vi "Teleop.vi"(10 "Match Info":T1={"Autonomous Elapsed Seconds"=0.0, "TeleOp Elapsed Seconds"=0.0, "Disabled Elapsed Seconds"=0.0, "Visited Autonomous"=FALSE, "Visited TeleOp"=FALSE, "Visited Disabled"=FALSE, "Autonomous Settings"={"Autonomous Style"=enum."Independent", "VI Refnum"=refnum}}, 11 "Call Context":T2) -> ()   [LabVIEW 2020]
doc: "This VI is called for each enabled TeleOp packet received from the DS. It is typically used to read from joysticks and other inputs and update I/O or setpoints for timed control loops. It should complete and return within 20 milliseconds or risk missing DS packets."
uses:
  <vilib>/Rock Robotics/WPI/DriverStation/WPI_DriverStationDerivedRobotMode.ctl
  <vilib>/Rock Robotics/WPI/DriverStation/WPI_DriverStationMatch Info.ctl
  Framework/Robot Global Data.vi
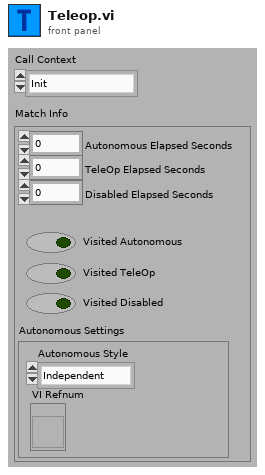
[diagram p1: front panel]
types:
  T1 = typedef "WPI_DriverStationMatch Info.ctl" = cluster{"Autonomous Elapsed Seconds":dbl, "TeleOp Elapsed Seconds":dbl, "Disabled Elapsed Seconds":dbl, "Visited Autonomous":bool, "Visited TeleOp":bool, "Visited Disabled":bool, "Autonomous Settings":cluster{"Autonomous Style":enum16{"Iterative", "Independent"}, "VI Refnum":refnum<vi>}}
  T2 = typedef "WPI_DriverStationDerivedRobotMode.ctl" = enum16{"Init", "Execute", "Stop"}
  T3 = typedef "Command Status Info.ctl" = cluster{"Name":string, "Status":T4, "notifier out":T5}
  T4 = typedef "Completion Status.ctl" = enum16{"Successful", "Aborted", "Incomplete"}
  T5 = typedef "Completion Notifier.ctl" = refnum<notifier>
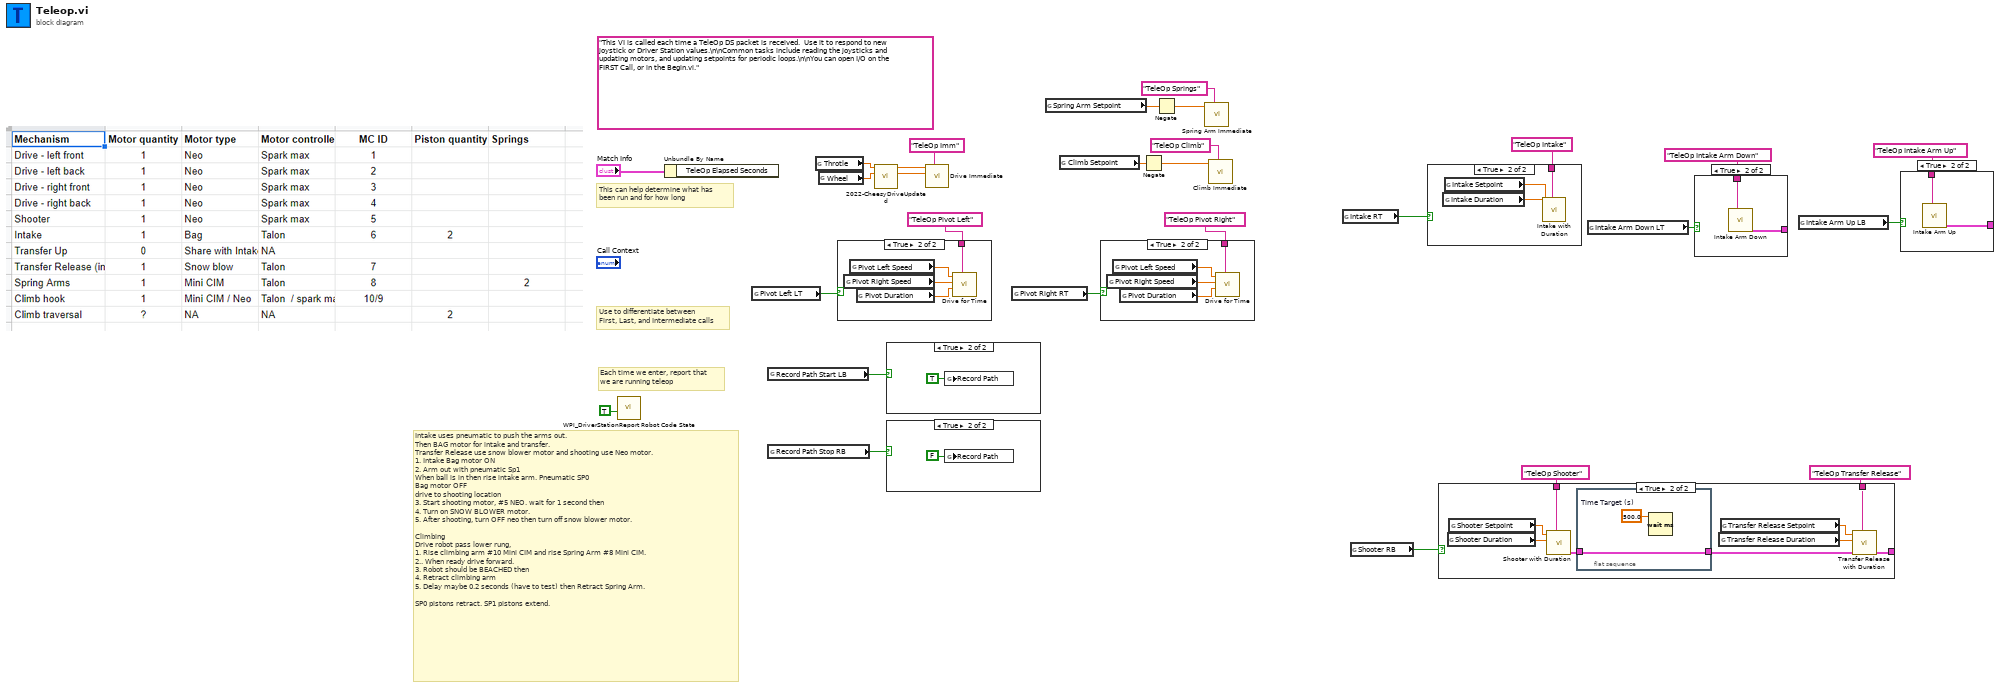
[diagram p0: block diagram]
diagram:
  (unwired) "This VI is called each time a TeleOp DS packet is received.  Use it to respond to new joystick or Driver Station values.\n\nCommon tasks include reading the joysticks and updating motors, and updating setpoints for periodic loops.\n\nYou can open I/O on the FIRST Call, or in the Begin.vi."
  # "Intake uses pneumatic to push the arms out. \nThen BAG motor for intake and transfer. \nTransfer Release use snow blower motor and shooting use Neo motor.\n1. Intake Bag motor ON\n2. Arm out with pneumatic Sp1\nWhen ball is in then rise intake arm. Pneumatic SP0\nBag motor OFF\ndrive to shooting location \n3. Start shooting motor, #5 NEO. wait for 1 second then\n4. Turn on SNOW BLOWER motor. \n5. After shooting, turn OFF neo then turn off snow blower motor.\n\nClimbing \nDrive robot pass lower rung, \n1. Rise climbing arm #10 Mini CIM and rise Spring Arm #8 Mini CIM. \n2.. When ready drive forward. \n3. Robot should be BEACHED then\n4. Retract climbing arm\n5. Delay maybe 0.2 seconds (have to test) then Retract Spring Arm.\n\nSP0 pistons retract. SP1 pistons extend."
  # "Each time we enter, report that\nwe are running teleop"
  # "Use to differentiate between\nFirst, Last, and Intermediate calls"
  # "This can help determine what has\nbeen run and for how long"
  n1 = call <vilib>:"WPI_DriverStationReport Robot Code State.vi"("TeleOp"=TRUE ("Autonomous")) -> ()  [unwired: 10 in, 1 out]
  n2 = Unbundle By Name("Match Info") -> ()  [unwired: 1 out]
  n3 = global read "Robot Global Data.vi" "Pivot Left LT"() -> (w5:bool)
  n4 = global read "Robot Global Data.vi" "Record Path Start LB"() -> (w2:bool)
  n5 = global read "Robot Global Data.vi" "Record Path Stop RB"() -> (w1:bool)
  n6 = global read "Robot Global Data.vi" "Throtle"() -> (w23:dbl)
  n7 = global read "Robot Global Data.vi" "Wheel"() -> (w22:dbl)
  n8 = case shown="True" w5 {
    tunnel: "TeleOp Pivot Left" ("Description") -> [_ w32]
    frame False {
    }
    frame True {
      n9 = global read "Robot Global Data.vi" "Pivot Right Speed"() -> (w30:dbl)
      n10 = global read "Robot Global Data.vi" "Pivot Left Speed"() -> (w31:dbl)
      n11 = global read "Robot Global Data.vi" "Pivot Duration"() -> (w29:dbl)
      n12 = call "Drive for Time.vi"("Description"=w32, "Seconds"=w29, "Right Speed"=w30, "Left Speed"=w31) -> ()  [unwired: 7 in, 1 out]
    }
  }
  n13 = call "2022-CheesyDriveUpdated.vi"("Throttle"=w23, "Wheel"=w22) -> ("Left PWM"=w25:dbl, "Right PWM"=w24:dbl)  [unwired: 11 in, 1 out]
  n14 = case shown="True" w2 {
    frame False {
    }
    frame True {
      n15 = global write "Robot Global Data.vi" "Record Path"(TRUE ("Record Path")) -> ()
    }
  }
  n16 = case shown="True" w1 {
    frame False {
    }
    frame True {
      n17 = global write "Robot Global Data.vi" "Record Path"(FALSE ("Record Path")) -> ()
    }
  }
  n18 = call "Drive Immediate.vi"("Description"="TeleOp Imm", "Right Setpoint"=w24, "Left Setpoint"=w25) -> ()  [unwired: 8 in, 1 out]
  n19 = global read "Robot Global Data.vi" "Pivot Right RT"() -> (w4:bool)
  n20 = global read "Robot Global Data.vi" "Spring Arm Setpoint"() -> (w12:dbl)
  n21 = global read "Robot Global Data.vi" "Climb Setpoint"() -> (w15:dbl)
  n22 = case shown="True" w4 {
    tunnel: "TeleOp Pivot Right" ("Description") -> [_ w38]
    frame False {
    }
    frame True {
      n23 = global read "Robot Global Data.vi" "Pivot Right Speed"() -> (w36:dbl)
      n24 = global read "Robot Global Data.vi" "Pivot Left Speed"() -> (w37:dbl)
      n25 = global read "Robot Global Data.vi" "Pivot Duration"() -> (w35:dbl)
      n26 = call "Drive for Time.vi"("Description"=w38, "Seconds"=w35, "Right Speed"=w36, "Left Speed"=w37) -> ()  [unwired: 7 in, 1 out]
    }
  }
  n27 = Negate(x=w15) -> (-x=w11:dbl)
  n28 = Negate(x=w12) -> (-x=w10:dbl)
  n29 = call "Spring Arm Immediate.vi"("Description"="TeleOp Springs", "Setpoint"=w10) -> ()  [unwired: 9 in, 1 out]
  n30 = call "Climb Immediate.vi"("Description"="TeleOp Climb", "Setpoint"=w11) -> ()  [unwired: 9 in, 1 out]
  n31 = global read "Robot Global Data.vi" "Intake RT"() -> (w21:bool)
  n32 = global read "Robot Global Data.vi" "Shooter RB"() -> (w9:bool)
  n33 = case shown="True" w21 {
    tunnel: "TeleOp Intake" ("Description") -> [_ w41]
    frame False {
    }
    frame True {
      n34 = global read "Robot Global Data.vi" "Intake Duration"() -> (w39:dbl)
      n35 = global read "Robot Global Data.vi" "Intake Setpoint"() -> (w40:dbl)
      n36 = call "Intake with Duration.vi"("Description"=w41, "Duration (s)"=w39, "Setpoint"=w40) -> ()  [unwired: 8 in, 1 out]
    }
  }
  n37 = case shown="True" w9 {
    tunnel: "TeleOp Shooter" ("Description") -> [_ w50]
    tunnel: [_ w47] -> _
    tunnel: "TeleOp Transfer Release" ("Description") -> [_ w46]
    frame False {
    }
    frame True {
      n38 = global read "Robot Global Data.vi" "Shooter Duration"() -> (w48:dbl)
      n39 = global read "Robot Global Data.vi" "Shooter Setpoint"() -> (w49:dbl)
      n40 = call "Shooter with Duration.vi"("Description"=w50, "Duration (s)"=w48, "Setpoint"=w49) -> ("Command Info Out"=w43:T3)  [unwired: 8 in]
      n41 = flat-sequence {
        tunnel: [w51] -> w42
        tunnel: w43 -> [w51]
        frame #0 {
          w52 = 500.0  # Time Target (s)
          n42 = Wait (ms)(milliseconds to wait=w52) -> ()  [unwired: 1 out]
        }
      }
      n43 = global read "Robot Global Data.vi" "Transfer Release Duration"() -> (w45:dbl)
      n44 = global read "Robot Global Data.vi" "Transfer Release Setpoint"() -> (w44:dbl)
      n45 = call "Transfer Release with Duration.vi"("Description"=w46, "Command Info In"=w42, "Duration (s)"=w45, "Setpoint"=w44) -> ("Command Info Out"=w47:T3)  [unwired: 7 in]
    }
  }
  n46 = global read "Robot Global Data.vi" "Intake Arm Down LT"() -> (w19:bool)
  n47 = case shown="True" w19 {
    tunnel: "TeleOp Intake Arm Down" ("Description") -> [_ w54]
    tunnel: [_ w53] -> _
    frame False {
    }
    frame True {
      n48 = call "Intake Arm Down.vi"("Description"=w54) -> ("Command Info Out"=w53:T3)  [unwired: 10 in]
    }
  }
  n49 = global read "Robot Global Data.vi" "Intake Arm Up LB"() -> (w16:bool)
  n50 = case shown="True" w16 {
    tunnel: [_ w56] -> _
    tunnel: "TeleOp Intake Arm Up" ("Description") -> [_ w55]
    frame False {
    }
    frame True {
      n51 = call "Intake Arm Up.vi"("Description"=w55) -> ("Command Info Out"=w56:T3)  [unwired: 10 in]
    }
  }
